vi "grSim Packet Command UDP Test.vi"(7 "replace ball":bool, 8 "Port:":u16=20011, 9 "SSL Vision Address:":string="127.0.0.1", 10 "isteamyellow":bool=TRUE, 11 "Robots":T4[](array[typedef])) -> ()   [LabVIEW 2017]
uses:
  grSim Robot Command.ctl
  grSim RobotReplacement.ctl
  grSim_BallReplacement.ctl
panel:
  in  "grSim replacement":T3={"grSim_RobotReplacement"=[{"x"=0.0, "y"=-450.0, "dir"=0.0, "yellowteam"=FALSE, "id"=0}, {"x"=0.0, "y"=-270.0, "dir"=0.0, "yellowteam"=FALSE, "id"=1}, {"x"=0.0, "y"=-90.0, "dir"=0.0, "yellowteam"=FALSE, "id"=2}, {"x"=0.0, "y"=90.0, "dir"=0.0, "yellowteam"=FALSE, "id"=3}, {"x"=0.0, "y"=270.0, "dir"=0.0, "yellowteam"=FALSE, "id"=4}, {"x"=0.0, "y"=450.0, "dir"=0.0, "yellowteam"=FALSE, "id"=5}], "grSim_BallReplacement"={"x"=0.0, "y"=0.0, "vx"=0.0, "vy"=0.0}}
  out "error out":errorcluster
  out "Array":u8[](array[numeric]) format="%02x"
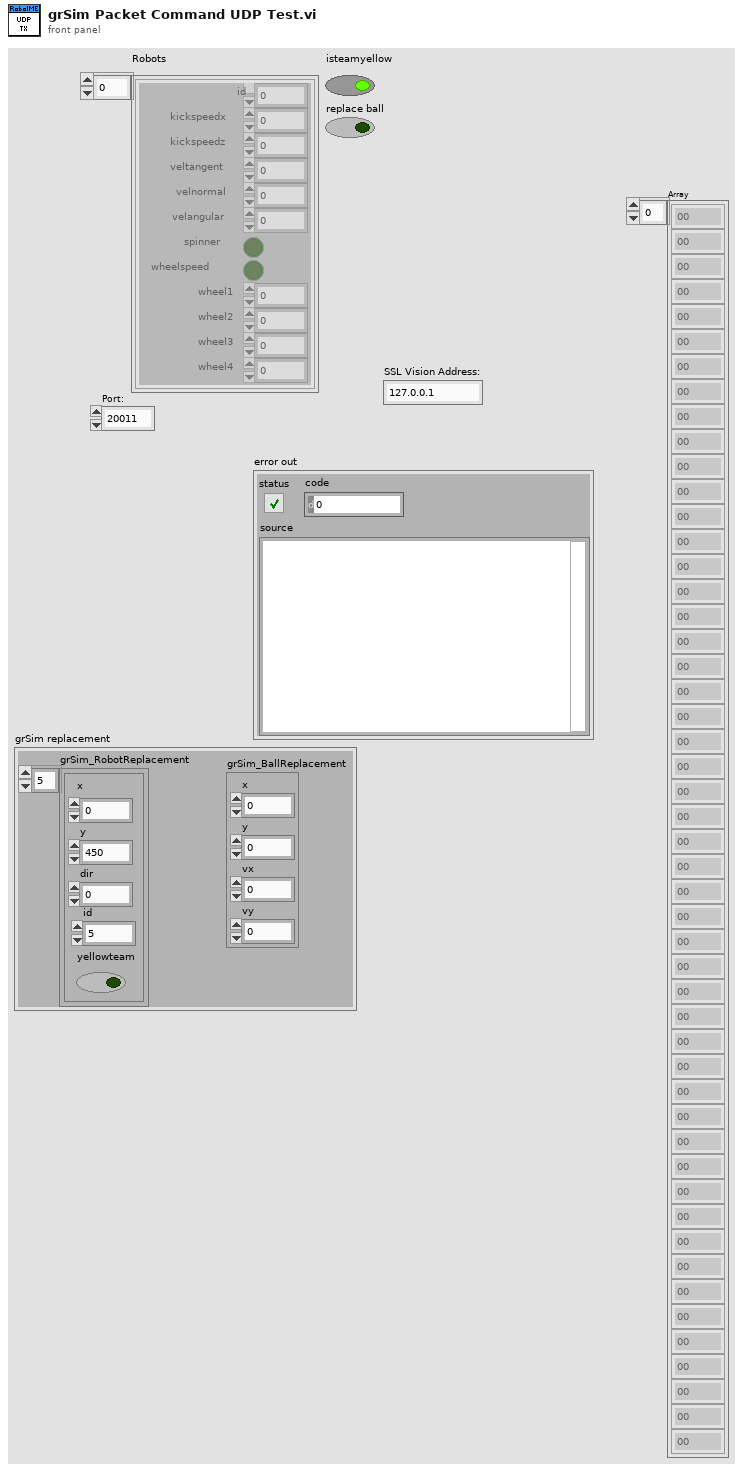
[diagram p1: front panel]
types:
  T1 = typedef "grSim RobotReplacement.ctl" = cluster{"x":dbl, "y":dbl, "dir":dbl, "yellowteam":bool, "id":u32}
  T2 = typedef "grSim_BallReplacement.ctl" = cluster{"x":dbl, "y":dbl, "vx":dbl, "vy":dbl}
  T3 = cluster{"grSim_RobotReplacement":T1[], "grSim_BallReplacement":T2}
  T4 = typedef "grSim Robot Command.ctl" = cluster{"id":u32, "kickspeedx":sgl, "kickspeedz":sgl, "veltangent":sgl, "velnormal":sgl, "velangular":sgl, "spinner":bool, "wheelspeed":bool, "wheel1":sgl, "wheel2":sgl, "wheel3":sgl, "wheel4":sgl}
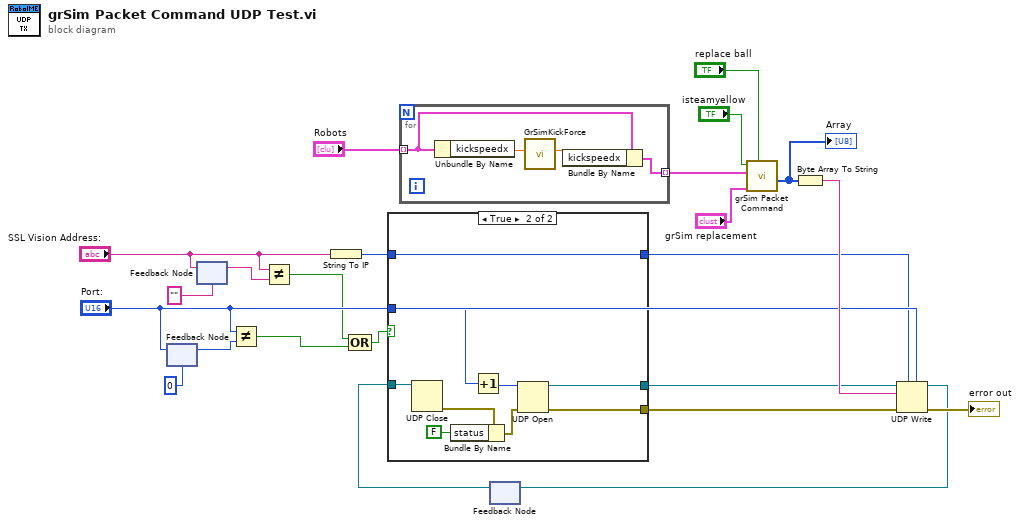
[diagram p0: block diagram]
diagram:
  n1 = feedback #1(u16 0 ("Port:")) -> (w19:u16)
  n2 = feedback-in #1("Port:") -> ()
  n3 = feedback #2("" ("SSL Vision Address:")) -> (w17:string)
  n4 = feedback-in #2("SSL Vision Address:") -> ()
  n5 = Not Equal?(x="Port:", y=w19) -> (x != y?=w15:bool)
  n6 = Not Equal?(x="SSL Vision Address:", y=w17) -> (x != y?=w16:bool)
  n7 = String To IP(1:"SSL Vision Address:") -> (0:w6:u32)
  n8 = Compound Arithmetic op=OR(w16, w15) -> (w14:bool)
  n9 = for {
    tunnel: "Robots" -> [w27] mode=indexing
    tunnel: [w26] -> w3 mode=indexing
    n10 = Unbundle By Name(w27) -> ("kickspeedx"=w25:sgl)
    n11 = call "GrSimKickForce.vi"("real kick"=w25) -> ("grsim kick"=w24:dbl)  [unwired: 10 in]
    n12 = Bundle By Name(cluster=w27, "kickspeedx"=w24) -> (w26:T4)
  }
  n13 = feedback #3() -> (w12:refnum<k16>)  [unwired: 1 in]
  n14 = case shown="True" w14 {
    tunnel: [_ w38] -> w20
    tunnel: [w29 w36] -> w11
    tunnel: "Port:" -> [_ w35]
    tunnel: w6 -> [w28 w33]
    tunnel: w12 -> [w29 w34]
    tunnel: [w28 w33] -> w5
    frame False {
    }
    frame True {
      n15 = UDP Close(connection ID=w34) -> (error out=w32:errorcluster)  [unwired: 1 in, 1 out]
      n16 = Bundle By Name(cluster=w32, "status"=FALSE) -> (w31:errorcluster)
      n17 = Increment(x=w35) -> (x+1=w37:u16)
      n18 = UDP Open(8:w31, 11:w37) -> (port=w36:refnum<k16>, 0:w38:errorcluster)  [unwired: 3 in, 1 out]
    }
  }
  n19 = call "grSim Packet Command.vi"("replace ball"="replace ball", "grSim replacement"="grSim replacement", "Robots"=w3, "isteamyellow"="isteamyellow") -> ("Array"=w22:u8[])  [unwired: 7 in]
  "Array" <- w22
  n20 = Byte Array To String(unsigned byte array=w22) -> (string=w21:string)
  n21 = UDP Write(address=w5, port or service name="Port:", connection ID=w11, data in=w21, 8:w20) -> (error out=→"error out":errorcluster, 3:w10:refnum<k16>)  [unwired: 1 in]
  n22 = feedback-in #3(w10) -> ()
